vi "Write Data.vi"(8 "error in (no error)":errorcluster, 9 "Publication Time":timestamp, 10 "Value":variant, 11 "TerminalReference in":refnum<class "TerminalReference.lvclass">) -> (0 "error out":errorcluster, 3 "TerminalReference out":refnum<class "TerminalReference.lvclass">)   [LabVIEW 2015, in "Mediator.lvlib" / "TerminalReference.lvclass"]
uses:
  TerminalReference.lvclass
  TerminalReference.lvclass/TerminalReference.ctl
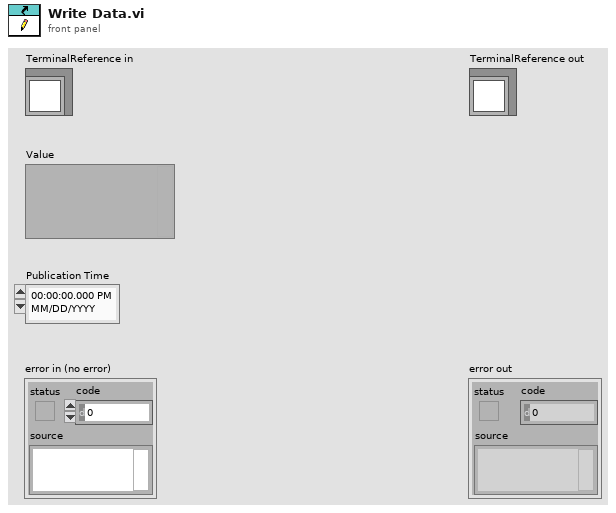
[diagram p1: front panel]
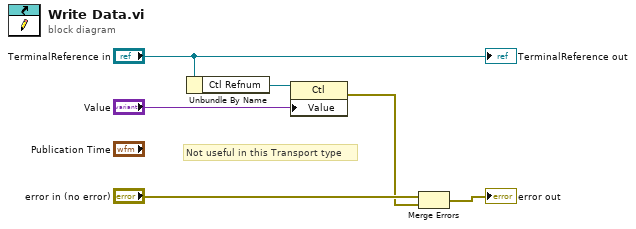
[diagram p0: block diagram]
diagram:
  # "Not useful in this Transport type"
  n1 = Unbundle By Name("TerminalReference in") -> ("Ctl Refnum"=w4:refnum<vi>)
  n2 = property class="Ctl"(reference=w4, "Value"="Value") -> (error out=w1:errorcluster)  [unwired: 1 in, 1 out]
  n3 = Merge Errors("error in (no error)", w1) -> (→"error out":errorcluster)
  "TerminalReference out" <- "TerminalReference in"
